vi "Get Wind Dir Calibration Offset V.vi"(8 "error in (no error)":errorcluster, 11 "windDirCal":i16) -> (0 "error out":errorcluster, 2 "function return":i32, 3 "windDirCal out":i16)   [LabVIEW 2009, in "VantagePro.lvlib"]
doc: "DllAccess int _stdcall GetWindDirCalibrationOffset_V( short &windDirCal );"
uses:
  VantagePro.lvlib
  <userlib>/VantagePro/VantagePro.dll
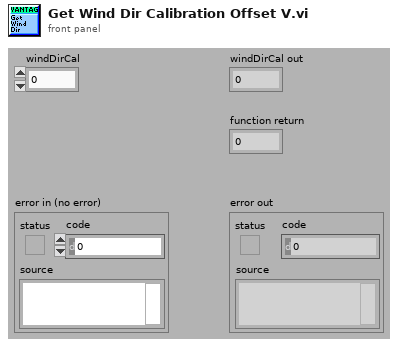
[diagram p1: front panel]
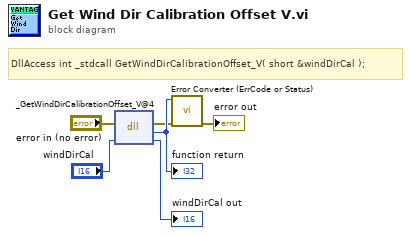
[diagram p0: block diagram]
diagram:
  # "DllAccess int _stdcall GetWindDirCalibrationOffset_V( short &windDirCal );"
  n1 = dll-call lib="C:/Program Files/National Instruments/LabVIEW 2010/user.lib/VantagePro/VantagePro.*" fn="_GetWindDirCalibrationOffset_V@4"(error in="error in (no error)", "windDirCal"="windDirCal") -> (error out=w2:errorcluster, w6:i32, "windDirCal"=→"windDirCal out":i16)  [unwired: 2 in, 1 out]
  "function return" <- w6
  n2 = call "Error Converter (ErrCode or Status).vi"("error in (no error)"=w2, "error code"=w6) -> ("error out"=→"error out":errorcluster)  [unwired: 9 in]
